vi "MH_WRabbitInitLink.vi"(8 "error in (no error)":errorcluster, 10 "link_on":i32, 11 "devidx":i32) -> (0 "error out":errorcluster, 3 "return type":i32)   [LabVIEW 2019]
uses:
  MH_DllPath_global.vi
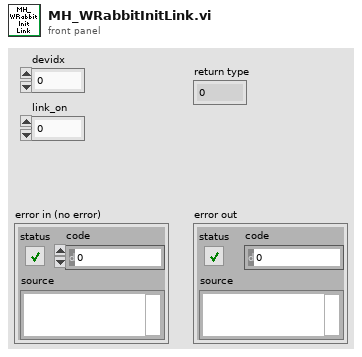
[diagram p1: front panel]
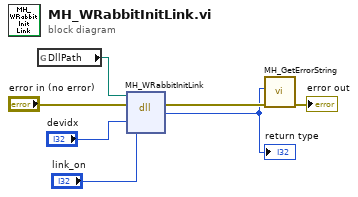
[diagram p0: block diagram]
diagram:
  n1 = global read "MH_DllPath_global.vi" "DllPath"() -> (w6:path)
  n2 = dll-call lib="MHLib64.dll" fn="MH_WRabbitInitLink"(path in=w6, error in="error in (no error)", "devidx"="devidx", "link_on"="link_on") -> (error out=w5:errorcluster, "return type"=w2:i32)  [unwired: 3 in, 1 out]
  "return type" <- w2
  n3 = call "MH_GetErrorString.vi"("error in (no error)"=w5, "code"=w2) -> ("error out"=→"error out":errorcluster)  [unwired: 7 in, 2 out]
